vi "ofdm_qian.vi"() -> ()   [LabVIEW 2024]
panel:
  out "rate":dbl[](array[numeric])
  out "XY Graph 11":cluster{"Y":dbl[], "Y":dbl[]}[](graph) caption="多径"
  out "XY Graph 10":cluster{"Y":dbl[], "Y":dbl[]}[](graph) caption="单径"
  out "i_mult":dbl[](array[numeric])
  out "r_mult":dbl[](array[numeric])
  out "i_single":dbl[](array[numeric])
  out "r_single":dbl[](array[numeric])
  out "XY Graph 9":cluster{"Y":dbl[], "Y":dbl[]}[](graph) caption="加窗频谱"
  out "y_nowin":dbl[](array[numeric])
  out "XY Graph 8":cluster{"Y":dbl[], "Y":dbl[]}[](graph) caption="未加窗频谱"
  out "orgin_aver_power1":dbl[](array[numeric])
  out "y_win":dbl[](array[numeric])
  out "x_win":dbl[](array[numeric])
  out "orgin_aver_power":dbl[](array[numeric])
  out "x_nowin":dbl[](array[numeric])
  out "t_single":dbl[](array[numeric])
  out "signal_Tx":dbl[](array[numeric])
  out "t_mult":dbl[](array[numeric])
  out "signal_Tx_mult":dbl[](array[numeric])
  out "XY Graph 7":cluster{"Y":dbl[], "Y":dbl[]}[](graph) caption="多径"
  out "XY Graph 6":cluster{"Y":dbl[], "Y":dbl[]}[](graph) caption="单径"
  out "XY Graph 5":cluster{"Y":dbl[], "Y":dbl[]}[](graph) caption="单个ofdm符号+窗"
  out "A_window":dbl[](array[numeric])
  out "t_window":dbl[](array[numeric])
  in  "alpha":dbl
  out "XY Graph 4":cluster{"Y":dbl[], "Y":dbl[]}[](graph) caption="单个ofdm符号+cp+cs"
  out "A_cp":dbl[](array[numeric])
  out "t_cp":dbl[](array[numeric])
  in  "CS_length":u32
  in  "CP_length":u32
  out "XY Graph 3":cluster{"Y":dbl[], "Y":dbl[]}[](graph) caption="单个ofdm符号时域图"
  out "t":dbl[](array[numeric])
  out "A":dbl[](array[numeric])
  out "y":dbl[](array[numeric])
  out "x":dbl[](array[numeric])
  out "size(bit_moded)":dbl
  out "XY Graph 2":cluster{"Y":dbl[], "Y":dbl[]}[](graph) caption="第一个ofdm符号子载波幅度"
  in  "ifft_length":dbl
  out "i":dbl[](array[numeric])
  out "r":dbl[](array[numeric])
  out "size(bit_sequence)":dbl
  out "bit_sequence":i32[](array[numeric])
  out "bit_length":dbl
  out "XY Graph":cluster{"Y":dbl[], "Y":dbl[]}[](graph) caption="QAM调制散点图"
  in  "symbol_count":u32
  in  "bit_per_symbol":u32
  in  "carrier_count":u32
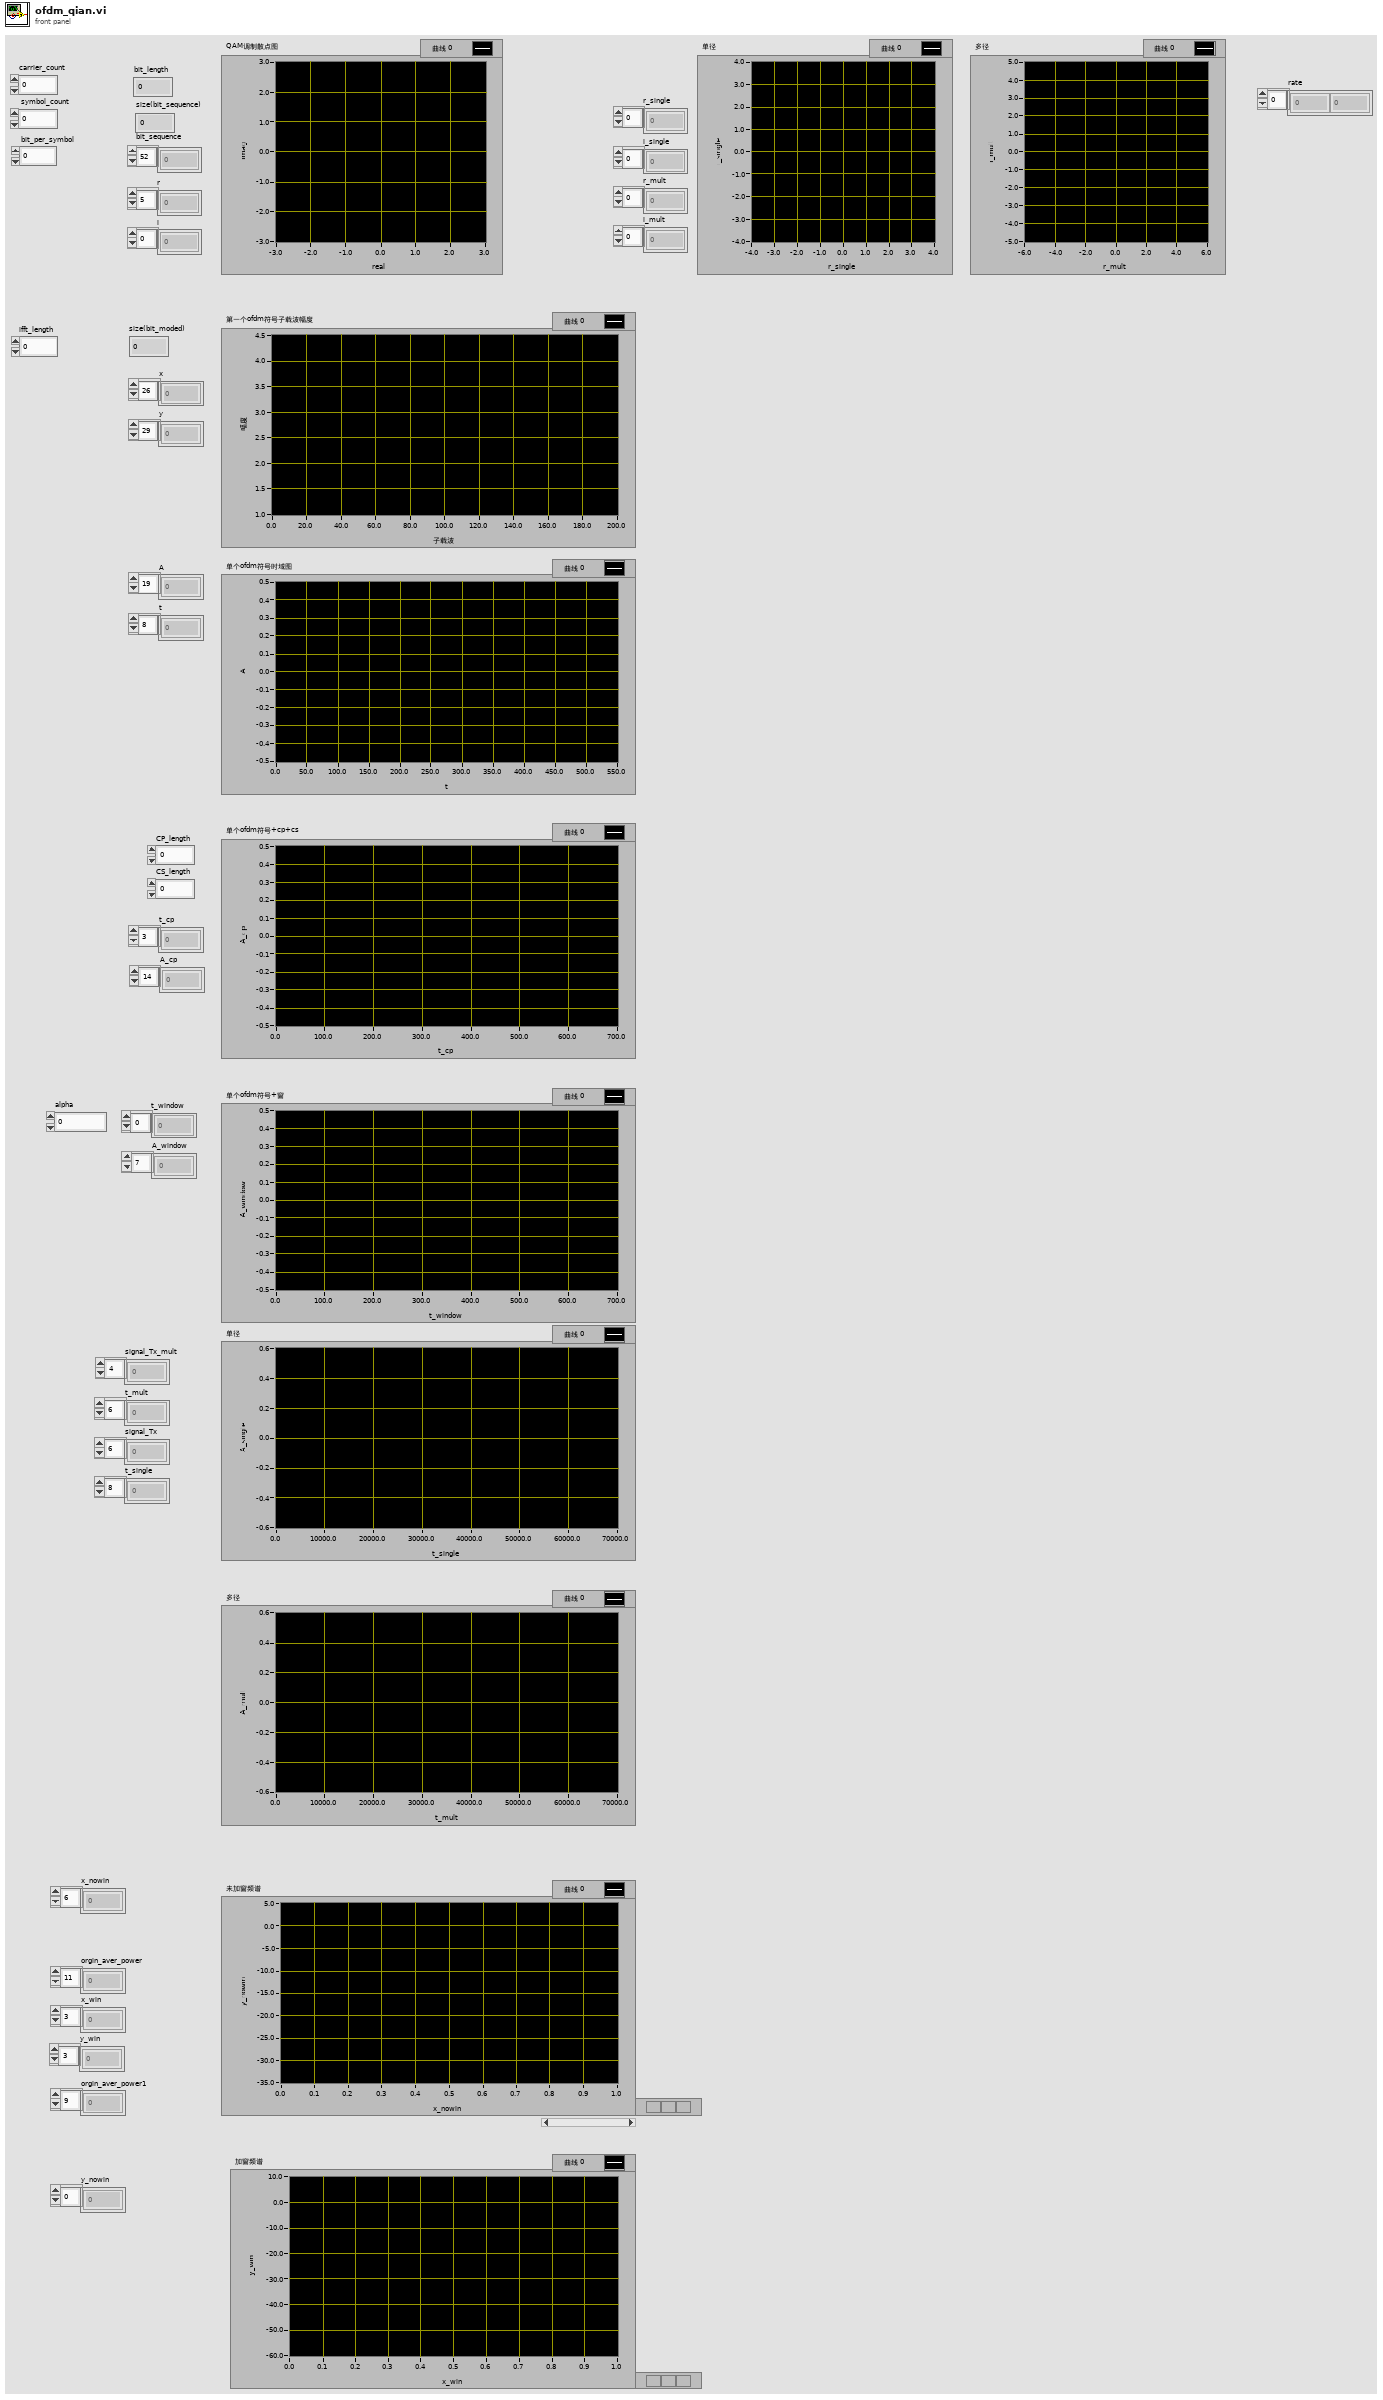
[diagram p1: front panel]
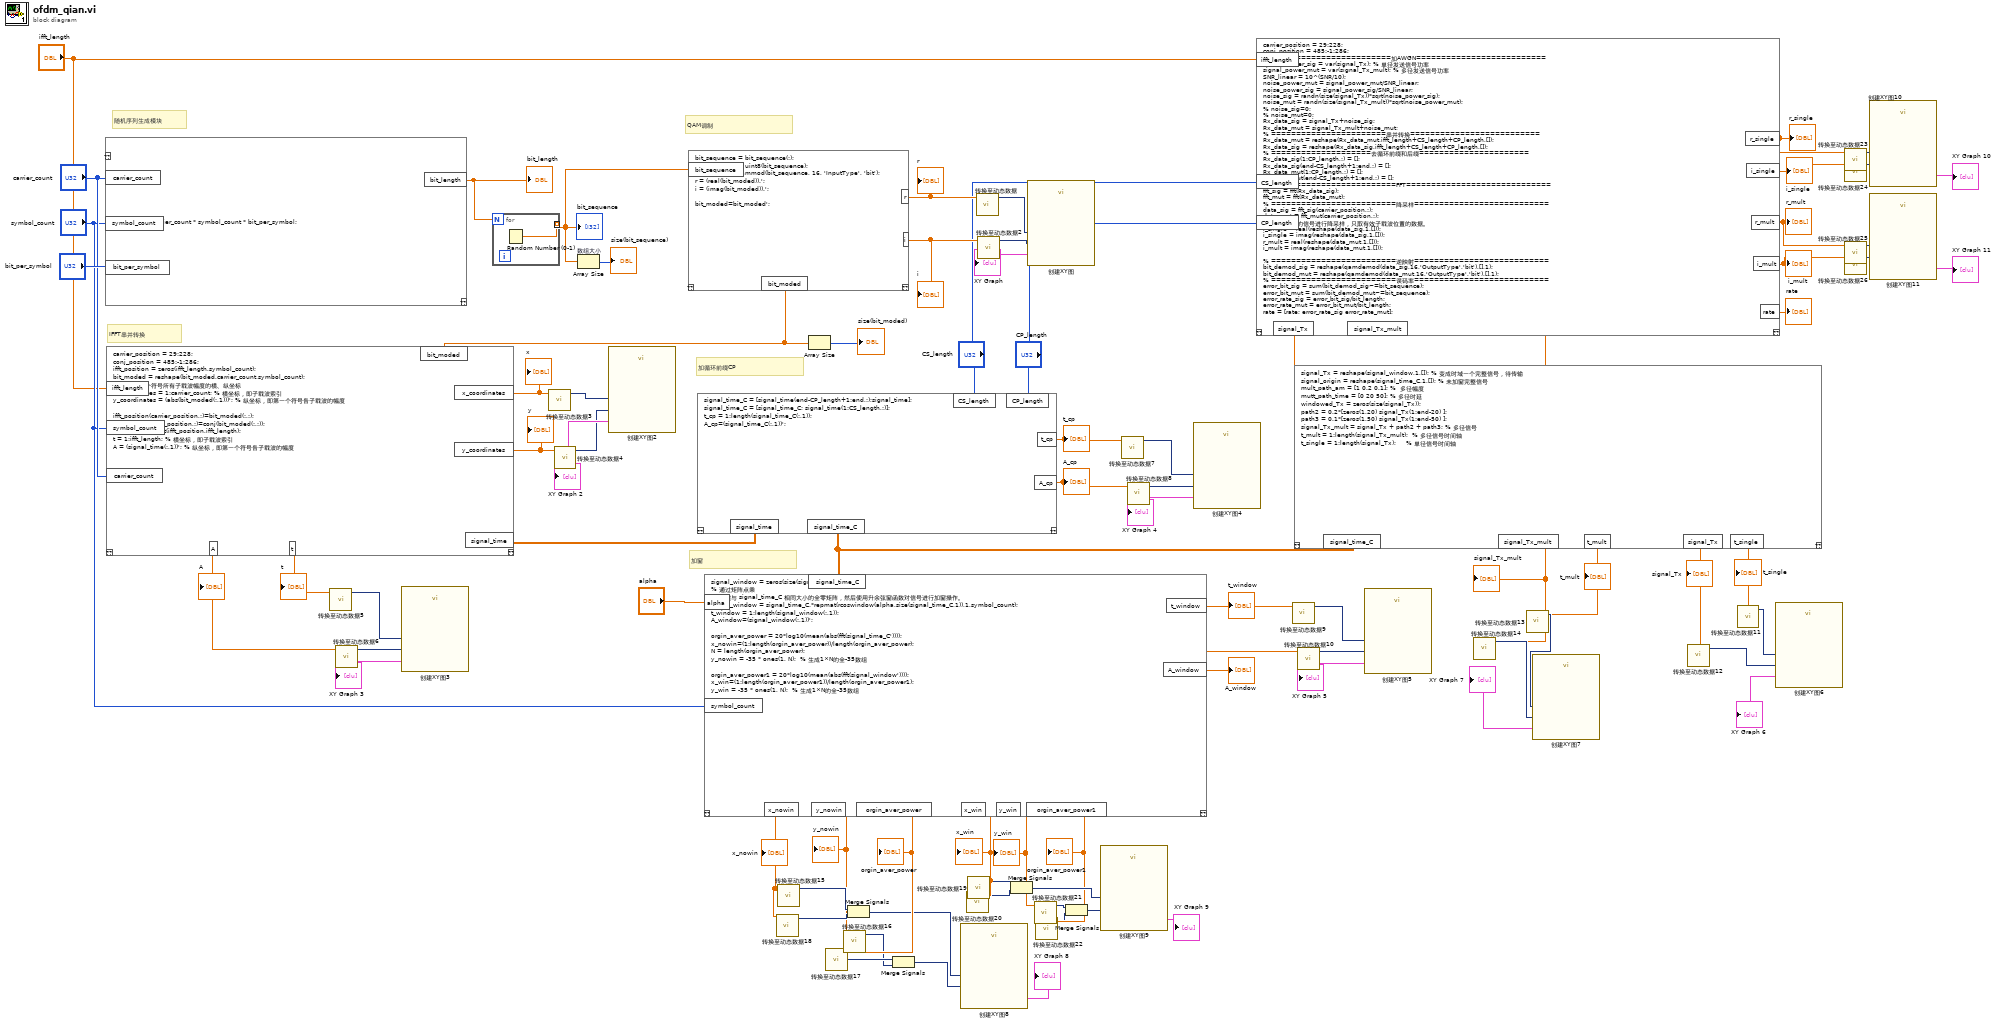
[diagram p0: block diagram]
diagram:
  # "加窗"
  # "加循环前缀CP"
  # "IFFT串并转换"
  # "QAM调制"
  # "随机序列生成模块"
  n1 = script code="bit_length = carrier_count * symbol_count * bit_per_symbol;"("carrier_count"="carrier_count", "symbol_count"="symbol_count", "bit_per_symbol"="bit_per_symbol") -> ("bit_length"=w79:dbl)  [unwired: 1 in, 1 out]
  "bit_length" <- w79
  n2 = for {
    N: w79 -> [_]
    tunnel: [w81] -> w77 mode=indexing
    n3 = Random Number (0-1)() -> (number: 0 to 1=w81:dbl)
  }
  "bit_sequence" <- w77
  n4 = Array Size "数组大小"(array=w77) -> (size(s)=→"size(bit_sequence)":i32)
  n5 = script code="bit_sequence = bit_sequence(:);\nbit_sequence = uint8(bit_sequence);\nbit_moded = qammod(bit_sequence, 16, 'InputType', 'bit');\nr = (real(bit_moded)).';\ni = (imag(bit_moded)).';\n\nbit_moded=bit_moded';"("bit_sequence"=w77) -> ("r"=w73:dbl[], "i"=w72:dbl[], "bit_moded"=w70:cdb[])  [unwired: 1 in, 1 out]
  "r" <- w73
  "i" <- w72
  n6 = script code="carrier_position = 29:228;\nconj_position = 485:-1:286;\nifft_position = zeros(ifft_length,symbol_count);\nbit_moded = reshape(bit_moded,carrier_count,symbol_count);\n% 分离第一个符号所有子载波幅度的横、纵坐标\nx_coordinates = 1:carrier_count; % 横坐标，即子载波索引\ny_coordinates = (abs(bit_moded(:,1)))'; % 纵坐标，即第一个符号各子载波的幅度\n\nifft_position(carrier_position,:)=bit_moded(:,:);\nifft_position(conj_position,:)=conj(bit_moded(:,:));\nsignal_time = ifft(ifft_position,ifft_length);\nt = 1:ifft_length; % 横坐标，即子载波索引\nA = (signal_time(:,1))'; % 纵坐标，即第一个符号各子载波的幅度"("ifft_length"="ifft_length", "symbol_count"="symbol_count", "carrier_count"="carrier_count", "bit_moded"=w70) -> ("x_coordinates"=w65:dbl[], "y_coordinates"=w64:dbl[], "A"=w59:dbl[], "t"=w60:dbl[], "signal_time"=w58:dbl[][])  [unwired: 1 in, 1 out]
  "x" <- w65
  "y" <- w64
  "A" <- w59
  "t" <- w60
  n7 = call "转换至动态数据5"("Array"=w60) -> ("Dynamic Data Type"=w62:dynamicdata)  [unwired: 3 in]
  n8 = call "转换至动态数据6"("Array"=w59) -> ("Dynamic Data Type"=w61:dynamicdata)  [unwired: 3 in]
  n9 = call "创建XY图3"("Y Input"=w61, "X Input"=w62) -> ("XY Graph"=→"XY Graph 3":cluster{"X":dbl[], "Y":dbl[]}[])  [unwired: 8 in, 1 out]
  n10 = call "转换至动态数据3"("Array"=w65) -> ("Dynamic Data Type"=w67:dynamicdata)  [unwired: 3 in]
  n11 = call "转换至动态数据4"("Array"=w64) -> ("Dynamic Data Type"=w66:dynamicdata)  [unwired: 3 in]
  n12 = call "创建XY图2"("Y Input"=w66, "X Input"=w67) -> ("XY Graph"=→"XY Graph 2":cluster{"X":dbl[], "Y":dbl[]}[])  [unwired: 8 in, 1 out]
  n13 = script code="signal_time_C = [signal_time(end-CP_length+1:end,:);signal_time];\nsignal_time_C = [signal_time_C; signal_time(1:CS_length,:)];\nt_cp = 1:length(signal_time_C(:,1));\nA_cp=(signal_time_C(:,1))';"("CP_length"="CP_length", "signal_time"=w58, "CS_length"="CS_length") -> ("t_cp"=w54:dbl[], "A_cp"=w53:dbl[], "signal_time_C"=w45:dbl[][])  [unwired: 1 in, 1 out]
  "t_cp" <- w54
  "A_cp" <- w53
  n14 = script code="signal_window = zeros(size(signal_time_C));\n% 通过矩阵点乘\n% 创建与 signal_time_C 相同大小的全零矩阵，然后使用升余弦窗函数对信号进行加窗操作。\nsignal_window = signal_time_C.*repmat(rcoswindow(alpha,size(signal_time_C,1)),1,symbol_count);\nt_window = 1:length(signal_window(:,1));\nA_window=(signal_window(:,1))';\n\norgin_aver_power = 20*log10(mean(abs(fft(signal_time_C'))));\nx_nowin=(1:length(orgin_aver_power))/length(orgin_aver_power);\nN = length(orgin_aver_power);\ny_nowin = -35 * ones(1, N);  % 生成1×N的全-35数组\n\norgin_aver_power1 = 20*log10(mean(abs(fft(signal_window'))));\nx_win=(1:length(orgin_aver_power1))/length(orgin_aver_power1);\ny_win = -35 * ones(1, N);  % 生成1×N的全-35数组"("signal_time_C"=w45, "alpha"="alpha", "symbol_count"="symbol_count") -> ("t_window"=w47:dbl[], "A_window"=w46:dbl[], "x_nowin"=w31:dbl[], "y_nowin"=w27:dbl[], "orgin_aver_power"=w35:dbl[], "y_win"=w21:dbl[], "x_win"=w26:dbl[], "orgin_aver_power1"=w20:dbl[])  [unwired: 1 in, 1 out]
  "t_window" <- w47
  "A_window" <- w46
  "x_nowin" <- w31
  "orgin_aver_power" <- w35
  "x_win" <- w26
  "y_win" <- w21
  "orgin_aver_power1" <- w20
  "y_nowin" <- w27
  n15 = call "转换至动态数据18"("Array"=w31) -> ("Dynamic Data Type"=w29:dynamicdata)  [unwired: 3 in]
  n16 = call "转换至动态数据15"("Array"=w31) -> ("Dynamic Data Type"=w30:dynamicdata)  [unwired: 3 in]
  n17 = Array Size(array=w70) -> (size(s)=→"size(bit_moded)":i32)
  n18 = call "转换至动态数据17"("Array"=w35) -> ("Dynamic Data Type"=w34:dynamicdata)  [unwired: 3 in]
  n19 = call "转换至动态数据16"("Array"=w27) -> ("Dynamic Data Type"=w33:dynamicdata)  [unwired: 3 in]
  n20 = Merge Signals(w30, w29) -> (w28:dynamicdata)
  n21 = Merge Signals(w34, w33) -> (w32:dynamicdata)
  n22 = call "创建XY图8"("Y Input"=w32, "X Input"=w28) -> ("XY Graph"=→"XY Graph 8":cluster{"X":dbl[], "Y":dbl[]}[])  [unwired: 8 in, 1 out]
  n23 = call "转换至动态数据20"("Array"=w26) -> ("Dynamic Data Type"=w25:dynamicdata)  [unwired: 3 in]
  n24 = call "转换至动态数据19"("Array"=w26) -> ("Dynamic Data Type"=w24:dynamicdata)  [unwired: 3 in]
  n25 = call "转换至动态数据"("Array"=w73) -> ("Dynamic Data Type"=w75:dynamicdata)  [unwired: 3 in]
  n26 = call "转换至动态数据2"("Array"=w72) -> ("Dynamic Data Type"=w74:dynamicdata)  [unwired: 3 in]
  n27 = Merge Signals(w24, w25) -> (w22:dynamicdata)
  n28 = call "创建XY图"("Y Input"=w74, "X Input"=w75) -> ("XY Graph"=→"XY Graph":cluster{"X":dbl[], "Y":dbl[]}[])  [unwired: 8 in, 1 out]
  n29 = call "转换至动态数据21"("Array"=w21) -> ("Dynamic Data Type"=w19:dynamicdata)  [unwired: 3 in]
  n30 = call "转换至动态数据22"("Array"=w20) -> ("Dynamic Data Type"=w18:dynamicdata)  [unwired: 3 in]
  n31 = Merge Signals(w19, w18) -> (w17:dynamicdata)
  n32 = call "创建XY图9"("Y Input"=w17, "X Input"=w22) -> ("XY Graph"=→"XY Graph 9":cluster{"X":dbl[], "Y":dbl[]}[])  [unwired: 8 in, 1 out]
  n33 = call "转换至动态数据7"("Array"=w54) -> ("Dynamic Data Type"=w56:dynamicdata)  [unwired: 3 in]
  n34 = call "转换至动态数据8"("Array"=w53) -> ("Dynamic Data Type"=w55:dynamicdata)  [unwired: 3 in]
  n35 = call "创建XY图4"("Y Input"=w55, "X Input"=w56) -> ("XY Graph"=→"XY Graph 4":cluster{"X":dbl[], "Y":dbl[]}[])  [unwired: 8 in, 1 out]
  n36 = call "转换至动态数据9"("Array"=w47) -> ("Dynamic Data Type"=w49:dynamicdata)  [unwired: 3 in]
  n37 = script code="signal_Tx = reshape(signal_window,1,[]); % 变成时域一个完整信号，待传输\nsignal_origin = reshape(signal_time_C,1,[]); % 未加窗完整信号\nmult_path_am = [1 0.2 0.1]; %  多径幅度\nmutt_path_time = [0 20 50]; % 多径时延\nwindowed_Tx = zeros(size(signal_Tx));\npath2 = 0.2*[zeros(1,20) signal_Tx(1:end-20) ];\npath3 = 0.1*[zeros(1,50) signal_Tx(1:end-50) ];\nsignal_Tx_mult = signal_Tx + path2 + path3; % 多径信号\nt_mult = 1:length(signal_Tx_mult);  % 多径信号时间轴\nt_single = 1:length(signal_Tx);     % 单径信号时间轴"("signal_time_C"=w45) -> ("signal_Tx_mult"=w15:dbl[], "signal_Tx"=w16:dbl[], "t_mult"=w38:dbl[], "t_single"=w37:dbl[])  [unwired: 1 in, 1 out]
  "signal_Tx_mult" <- w15
  "t_mult" <- w38
  "signal_Tx" <- w16
  "t_single" <- w37
  n38 = script code="carrier_position = 29:228;\nconj_position = 485:-1:286;\n% ========================加AWGN==========================\nsignal_power_sig = var(signal_Tx); % 单径发送信号功率\nsignal_power_mut = var(signal_Tx_mult); % 多径发送信号功率\nSNR_linear = 10^(SNR/10);\nnoise_power_mut = signal_power_mut/SNR_linear;\nnoise_power_sig = signal_power_sig/SNR_linear;\nnoise_sig = randn(size(signal_Tx))*sqrt(noise_power_sig);\nnoise_mut = randn(size(signal_Tx_mult))*sqrt(noise_power_mut);\n% noise_sig=0;\n% noise_mut=0;\nRx_data_sig = signal_Tx+noise_sig;\nRx_data_mut = signal_Tx_mult+noise_mut;\n% =======================串并转换==========================\nRx_data_mut = reshape(Rx_data_mut,ifft_length+CS_length+CP_length,[]);\nRx_data_sig = reshape(Rx_data_sig,ifft_length+CS_length+CP_length,[]);\n% ====================去循环前缀和后缀======================\nRx_data_sig(1:CP_length,:) = [];\nRx_data_sig(end-CS_length+1:end,:) = [];\nRx_data_mut(1:CP_length,:) = [];\nRx_data_mut(end-CS_length+1:end,:) = [];\n% =========================FFT=============================\nfft_sig = fft(Rx_data_sig);\nfft_mut = fft(Rx_data_mut);\n% =========================降采样===========================\ndata_sig = fft_sig(carrier_position,:);\ndata_mut = fft_mut(carrier_position,:);\n% 对 FFT 后的信号进行降采样，只取有效子载波位置的数据。\nr_single = real(reshape(data_sig,1,[]));\ni_single = imag(reshape(data_sig,1,[]));\nr_mult = real(reshape(data_mut,1,[]));\ni_mult = imag(reshape(data_mut,1,[]));\n\n% =========================逆映射===========================\nbit_demod_sig = reshape(qamdemod(data_sig,16,'OutputType','bit'),[],1);\nbit_demod_mut = reshape(qamdemod(data_mut,16,'OutputType','bit'),[],1);\n% =========================误码率===========================\nerror_bit_sig = sum(bit_demod_sig~=bit_sequence);\nerror_bit_mut = sum(bit_demod_mut~=bit_sequence);\nerror_rate_sig = error_bit_sig/bit_length;\nerror_rate_mut = error_bit_mut/bit_length;\nrate = [rate; error_rate_sig error_rate_mut];"("signal_Tx"=w16, "signal_Tx_mult"=w15, "CP_length"="CP_length", "CS_length"="CS_length", "ifft_length"="ifft_length") -> ("r_single"=w9:dbl[], "i_single"=w7:dbl[], "r_mult"=w5:dbl[], "i_mult"=w3:dbl[], "rate"=→"rate":dbl[])  [unwired: 1 in, 1 out]
  "r_single" <- w9
  "i_single" <- w7
  "r_mult" <- w5
  "i_mult" <- w3
  n39 = call "转换至动态数据10"("Array"=w46) -> ("Dynamic Data Type"=w48:dynamicdata)  [unwired: 3 in]
  n40 = call "创建XY图5"("Y Input"=w48, "X Input"=w49) -> ("XY Graph"=→"XY Graph 5":cluster{"X":dbl[], "Y":dbl[]}[])  [unwired: 8 in, 1 out]
  n41 = call "转换至动态数据14"("Array"=w15) -> ("Dynamic Data Type"=w39:dynamicdata)  [unwired: 3 in]
  n42 = call "转换至动态数据13"("Array"=w38) -> ("Dynamic Data Type"=w40:dynamicdata)  [unwired: 3 in]
  n43 = call "创建XY图7"("Y Input"=w39, "X Input"=w40) -> ("XY Graph"=→"XY Graph 7":cluster{"X":dbl[], "Y":dbl[]}[])  [unwired: 8 in, 1 out]
  n44 = call "转换至动态数据12"("Array"=w16) -> ("Dynamic Data Type"=w42:dynamicdata)  [unwired: 3 in]
  n45 = call "转换至动态数据11"("Array"=w37) -> ("Dynamic Data Type"=w43:dynamicdata)  [unwired: 3 in]
  n46 = call "创建XY图6"("Y Input"=w42, "X Input"=w43) -> ("XY Graph"=→"XY Graph 6":cluster{"X":dbl[], "Y":dbl[]}[])  [unwired: 8 in, 1 out]
  n47 = call "转换至动态数据23"("Array"=w9) -> ("Dynamic Data Type"=w8:dynamicdata)  [unwired: 3 in]
  n48 = call "转换至动态数据24"("Array"=w7) -> ("Dynamic Data Type"=w6:dynamicdata)  [unwired: 3 in]
  n49 = call "转换至动态数据25"("Array"=w5) -> ("Dynamic Data Type"=w4:dynamicdata)  [unwired: 3 in]
  n50 = call "转换至动态数据26"("Array"=w3) -> ("Dynamic Data Type"=w2:dynamicdata)  [unwired: 3 in]
  n51 = call "创建XY图10"("Y Input"=w6, "X Input"=w8) -> ("XY Graph"=→"XY Graph 10":cluster{"X":dbl[], "Y":dbl[]}[])  [unwired: 8 in, 1 out]
  n52 = call "创建XY图11"("Y Input"=w2, "X Input"=w4) -> ("XY Graph"=→"XY Graph 11":cluster{"X":dbl[], "Y":dbl[]}[])  [unwired: 8 in, 1 out]
